vi "Shared - Stop.vi"(8 "error in (no error)":errorcluster caption="エラー入力（エラーなし）", 10 "Stop in":bool, 11 "FGV Mode":T1=enum."Get") -> (0 "error out":errorcluster caption="エラー出力", 2 "Stop out":bool)   [LabVIEW 2018]
uses:
  FGV Mode.ctl
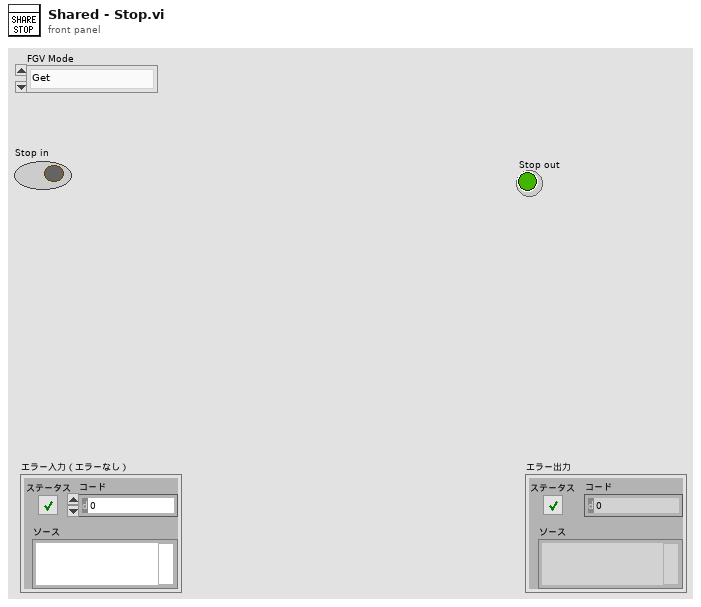
[diagram p1: front panel]
types:
  T1 = typedef "FGV Mode.ctl" = enum16{"None", "Init", "Set", "Get", "Update", "Clear"}
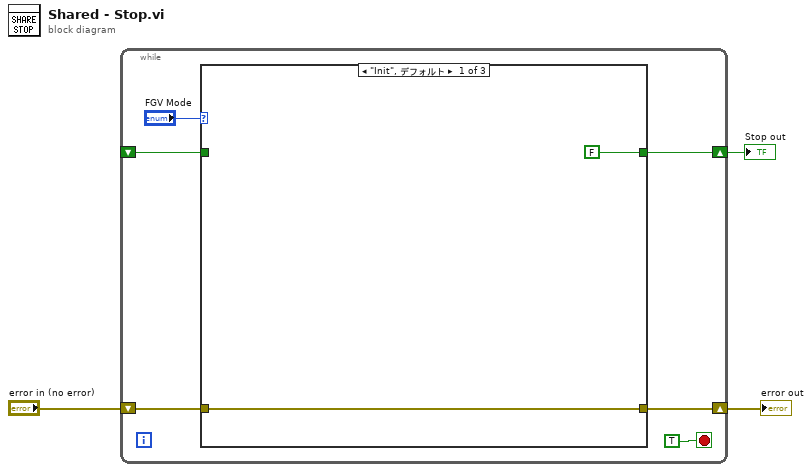
[diagram p0: block diagram]
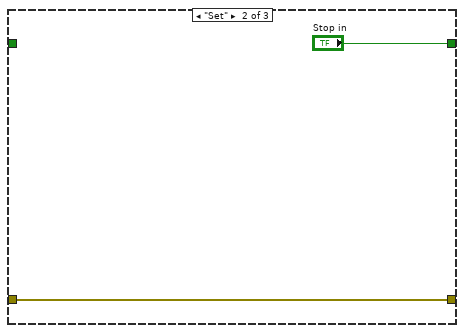
[diagram p2: hidden frame]
diagram:
  n1 = while {
    shift-right: [w7] -> w2
    shift-left: "error in (no error)" -> [w8]
    shift-right: [w5] -> w1
    shift-left: _ -> [w4]
    stop <- TRUE stop-if-true
    n2 = case shown="\"Init\", デフォルト" "FGV Mode" {
      tunnel: w8 -> [w11 w12 w14]
      tunnel: [w11 w12 w14] -> w7
      tunnel: [FALSE "Stop in" w15] -> w5
      tunnel: w4 -> [_ _ w15]
      frame "Init", Default {
      }
      frame "Set" {
      }
      frame "Get" {
      }
    }
  }
  "error out" <- w2
  "Stop out" <- w1
